vi "excel real time.vi"() -> ()   [LabVIEW 2022 SP3]
uses:
  <vilib>/Utility/NIReport.llb/Report Type.ctl
  <vilib>/Utility/NIReport.llb/Append Text Table to Report (wrap).vi
  <vilib>/Utility/NIReport.llb/NI_report.lvclass
  <vilib>/Utility/NIReport.llb/NI_ReportGenerationCore.lvlib
  <vilib>/Utility/NIReport.llb/Excel/NI_Excel.lvclass
panel:
  in  "report file path":path
  in  "stop":bool
  in  "Input 2":dbl
  in  "Input 1":dbl
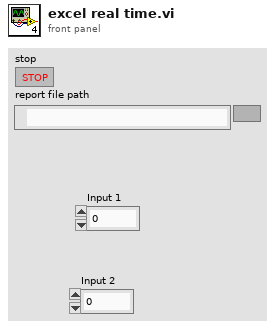
[diagram p1: front panel]
types:
  T1 = typedef "NI_ReportGenerationCore.lvlib/Report Type.ctl" = enum16{"HTML", "Word", "Excel"}
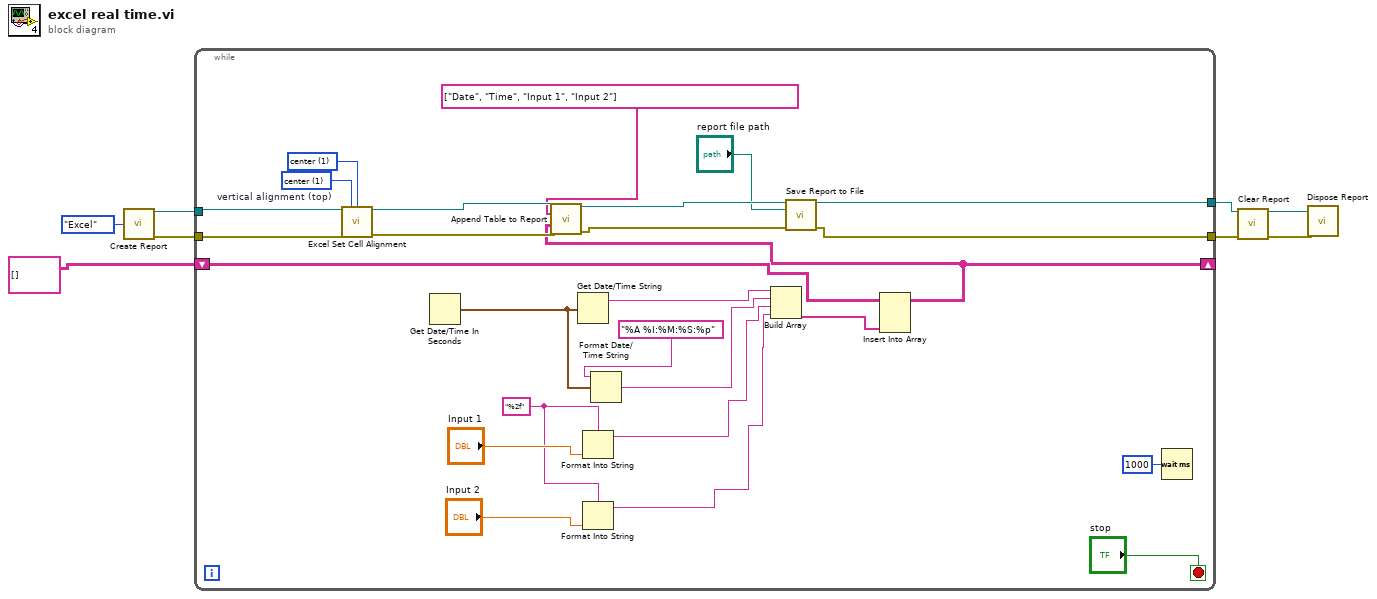
[diagram p0: block diagram]
diagram:
  n1 = call <vilib>:"Create Report.vi"("report type"=Report_Type."Excel") -> ("report out"=w7:refnum<class "NI_report.lvclass">, "error out"=w6:errorcluster)  [unwired: 13 in]
  n2 = while {
    tunnel: w7 -> [w32]
    tunnel: w6 -> [w31]
    tunnel: [w23] -> w5
    tunnel: [w22] -> w4
    shift-right: [w10] -> _
    shift-left: string[][] [] -> [w11]
    stop <- "stop" stop-if-true
    w15 = "%2f" ("format string")
    w29 = 1 items=["left", "center", "right"] ("horizontal alignment (left)")
    w30 = 1 items=["top", "center", "bottom"]  # vertical alignment (top)
    n3 = call <vilib>:"Excel Set Cell Alignment.vi"("report in"=w32, "vertical alignment (top)"=w30, "horizontal alignment (left)"=w29, "error in (no error)"=w31) -> ("report out"=w28:refnum<class "NI_report.lvclass">, "error out"=w27:errorcluster)  [unwired: 10 in]
    n4 = Get Date/Time In Seconds() -> (seconds since 1Jan1904=w21:timestamp)
    n5 = Get Date/Time String(seconds (now)=w21) -> (date string=w19:string)  [unwired: 2 in, 1 out]
    n6 = Format Into String(format string=w15, "Input 1") -> (resulting string=w14:string)  [unwired: 2 in, 1 out]
    n7 = Format Into String(format string=w15, "Input 2") -> (resulting string=w13:string)  [unwired: 2 in, 1 out]
    n8 = Format Date/Time String(time format string (%c)="%A %I:%M:%S:%p", seconds (now)=w21) -> (date/time string=w18:string)  [unwired: 1 in]
    n9 = Build Array(w19, w18, w14, w13) -> (w12:string[])
    n10 = Insert Into Array(array=w11, new element=w12) -> (w10:string[][])  [unwired: 2 in]
    n11 = call-poly <vilib>:"Append Table to Report.vi"("report in"=w28, "column headers"=string[] ["Date", "Time", "Input 1", "Input 2"], "text data"=w10, "error in (no error)"=w27) -> ("report out"=w25:refnum<class "NI_report.lvclass">, "error out"=w24:errorcluster)  [unwired: 8 in, 2 out]
    n12 = call-dynamic "Save Report to File.vi"("report in"=w25, "report file path"="report file path", "error in (no error)"=w24) -> ("report out"=w23:refnum<class "NI_report.lvclass">, "error out"=w22:errorcluster)  [unwired: 11 in]
    n13 = Wait (ms)(milliseconds to wait=u32 1000) -> ()  [unwired: 1 out]
  }
  n14 = call-dynamic "Clear Report.vi"("report in"=w5, "error in (no error)"=w4) -> ("report out"=w3:refnum<class "NI_report.lvclass">, "error out"=w2:errorcluster)  [unwired: 12 in]
  n15 = call-dynamic "Dispose Report.vi"("report in"=w3, "error in (no error)"=w2) -> ()  [unwired: 13 in, 1 out]
